vi "Vector3_ArbitraryRotate.vi"(1 "Arbitrary Axis (as UNIT Vector3)":dbl[](array[numeric])=[0.707107, -0.707107, 0.0], 2 "Input Vector3":dbl[](array[numeric])=[1.0, 0.0, 0.0], 3 "Rotation angle (deg)":dbl=90.0) -> (0 "Output Vector3":dbl[](array[numeric])=[0.5000003094490001, -0.500000309449, -0.707107])   [LabVIEW 2010]
uses:
  <vilib>/Analysis/baseanly.llb/Real Dot Product.vi
  <vilib>/Analysis/NI_AALBase.lvlib
panel:
  # "IMPORTANT NOTE:\n\nAxis of rotation must be a UNIT vector.\n\nAll rotations are CLOCKWISE looking INTO the axis of rotation."
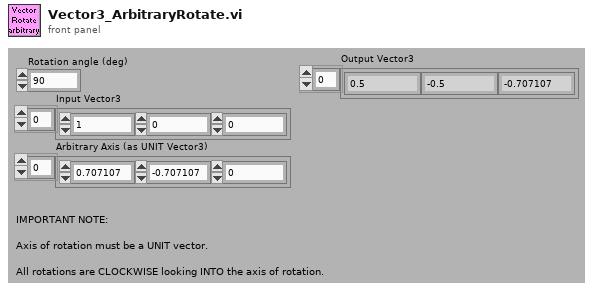
[diagram p1: front panel]
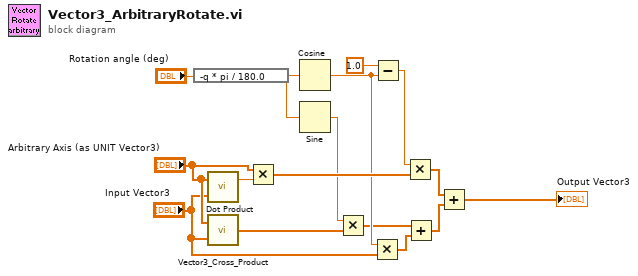
[diagram p0: block diagram]
diagram:
  n1 = expression code="-q * pi / 180.0"("Rotation angle (deg)") -> (w15:dbl)
  n2 = call-poly <vilib>:"Dot Product.vi"("Y Vector"="Input Vector3", "X Vector"="Arbitrary Axis (as UNIT Vector3)") -> ("X * Y"=w12:dbl)  [unwired: 1 out]
  n3 = call "Vector3_Cross_Product.vi"("V"="Input Vector3", "U"="Arbitrary Axis (as UNIT Vector3)") -> ("UxV"=w8:dbl[])
  n4 = Multiply(x="Arbitrary Axis (as UNIT Vector3)", y=w12) -> (x*y=w10:dbl[])
  n5 = Cosine(x=w15) -> (cos(x)=w6:dbl)
  n6 = Sine(x=w15) -> (sin(x)=w9:dbl)
  n7 = Multiply(x=w9, y=w8) -> (x*y=w4:dbl[])
  n8 = Multiply(x=w6, y="Input Vector3") -> (x*y=w5:dbl[])
  n9 = Subtract(x=1.0, y=w6) -> (x-y=w11:dbl)
  n10 = Multiply(x=w11, y=w10) -> (x*y=w2:dbl[])
  n11 = Add(x=w4, y=w5) -> (x+y=w3:dbl[])
  n12 = Add(x=w2, y=w3) -> (x+y=→"Output Vector3":dbl[])
